vi "FPGA_BIDIR_Sensores_dobles.vi"() -> ()   [LabVIEW 2015]
uses:
  <vilib>/LabVIEW Targets/FPGA/cRIO/shared/nicrio_ModuleControls/nicrio_cRIO-9234_DataRatesRing2.ctl
  <vilib>/LabVIEW Targets/FPGA/cRIO/shared/nicrio_ModuleControls/nicrio_BasicConversionTime.ctl
  <vilib>/rvi/Emulation/niFpgaGetClockAttributes.vi
  <vilib>/rvi/Emulation/niFpgaSctlEmulationGetInTimedLoop.vi
  <vilib>/rvi/Emulation/niFpgaEmulationReportErrorSimple.vi
  <vilib>/rvi/Emulation/niFpgaProcessEmulError.vi
  <vilib>/rvi/eio/common/nirviEmuTemplateMethod_errors.vi
  <vilib>/rvi/Emulation/niFpgaCriticalErrorInLSC.vi
  <vilib>/rvi/eio/common/nirviEmuTemplatePropertySet_errors.vi
  <vilib>/rvi/interface/RandomDataEmulation/niFpgaRandomDataHandleErrors.vi
  <vilib>/eio/EIONode/EIONode.xnode
  <vilib>/eio/EIOPropertyNode/EIOPropertyNode.xnode
  <vilib>/rvi/DataTransferAndStorage/Container/XNode/niFpgaContainer.xnode
  <vilib>/rvi/interface/RandomDataEmulation/nirviRandomDataFpgaReadWriteTemplate.vi
  <vilib>/rvi/eio/common/nirviEmuTemplatePropertyGet_errors.vi
  <vilib>/rvi/eio/common/nirviEmuTemplatePropertyGet_noerrors.vi
  <vilib>/rvi/eio/common/nirviEmuTemplatePropertySet_noerrors.vi
panel:
  out "Numeric 2":i32
  out "WhlCnt1":fxp<+/-,24,-4> format="%.27g"
  in  "Offset_WS1":fxp<+/-,24,-4>=0.000999998301267624 format="%.27g"
  out "Rueda1?":i16
  out "WhlCnt2":fxp<+/-,24,-4> format="%.27g"
  out "Rueda2?":i16
  out "RuedaDetectada1?":bool
  out "RuedaDetectada2?":bool
  out "Parar":bool
  out "Nº Ruedas 1":i32
  out "NºRuedas 2":i32
  in  "Offset_WS2":fxp<+/-,24,-4>=0.000999998301267624 format="%.27g"
  in  "Cycles to Filter":u16=5
  in  "Canal cero WS1?":bool=TRUE
  in  "Canal cero WS2?":bool=TRUE
  in  "Conversion Time":T1
  in  "Count(mSec)":u32=2
  in  "Stop":bool
  out "Buffer Underflow":bool
  in  "Digital?":bool=TRUE
  out "medidas":fxp<+/-,24,4>[](array[numeric])
  out "Buffer Overflow":bool
  out "Error Out":errorcluster
  in  "Data Rate":T2=2 items=["51.200 kS/s (NI 9234)"=1, "25.600 kS/s (NI 9234)"=2, "17.067 kS/s (NI 9234)"=3, "12.800 kS/s (NI 9234)"=4, "10.240 kS/s (NI 9234)"=5, "8.533 kS/s (NI 9234)"=6, "7.314 kS/s (NI 9234)"=7, "6.400 kS/s (NI 9234)"=8, "5.689 kS/s (NI 9234)"=9, "5.120 kS/s (NI 9234)"=10, "4.654 kS/s (NI 9234)"=11, "4.267 kS/s (NI 9234)"=12, "3.938 kS/s (NI 9234)"=13, "3.657 kS/s (NI 9234)"=14, "3.413 kS/s (NI 9234)"=15, "3.200 kS/s (NI 9234)"=16, "3.012 kS/s (NI 9234)"=17, "2.845 kS/s (NI 9234)"=18, "2.695 kS/s (NI 9234)"=19, "2.560 kS/s (NI 9234)"=20, "2.438 kS/s (NI 9234)"=21, "2.328 kS/s (NI 9234)"=22, "2.226 kS/s (NI 9234)"=23, "2.133 kS/s (NI 9234)"=24, "2.048 kS/s (NI 9234)"=25, "1.969 kS/s (NI 9234)"=26, "1.896 kS/s (NI 9234)"=27, "1.829 kS/s (NI 9234)"=28, "1.765 kS/s (NI 9234)"=29, "1.707 kS/s (NI 9234)"=30, "1.652 kS/s (NI 9234)"=31]
  out "DC OK":bool
  in  "Fotocélula":bool
  out "Detector de\npresencia":bool
  out "Chassis Temperature":i16
  out "Direccion 0?":bool
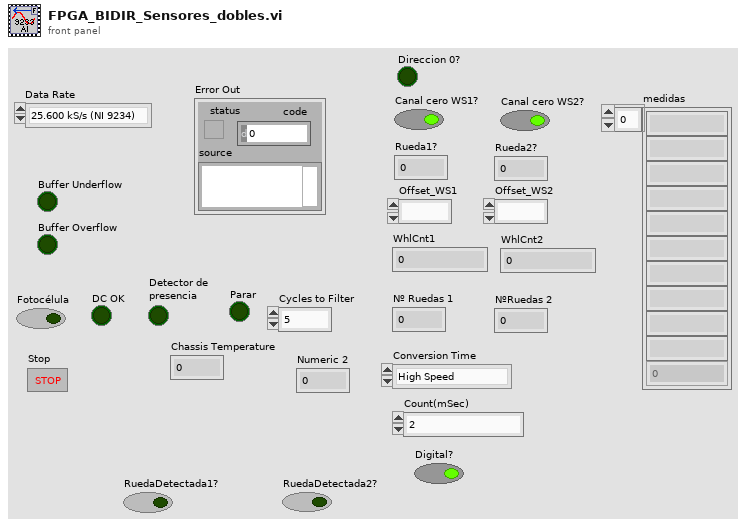
[diagram p1: front panel]
types:
  T1 = typedef "nicrio_BasicConversionTime.ctl" = enum8{"High Speed", "High Resolution"}
  T2 = typedef "nicrio_cRIO-9234_DataRatesRing2.ctl" = u8
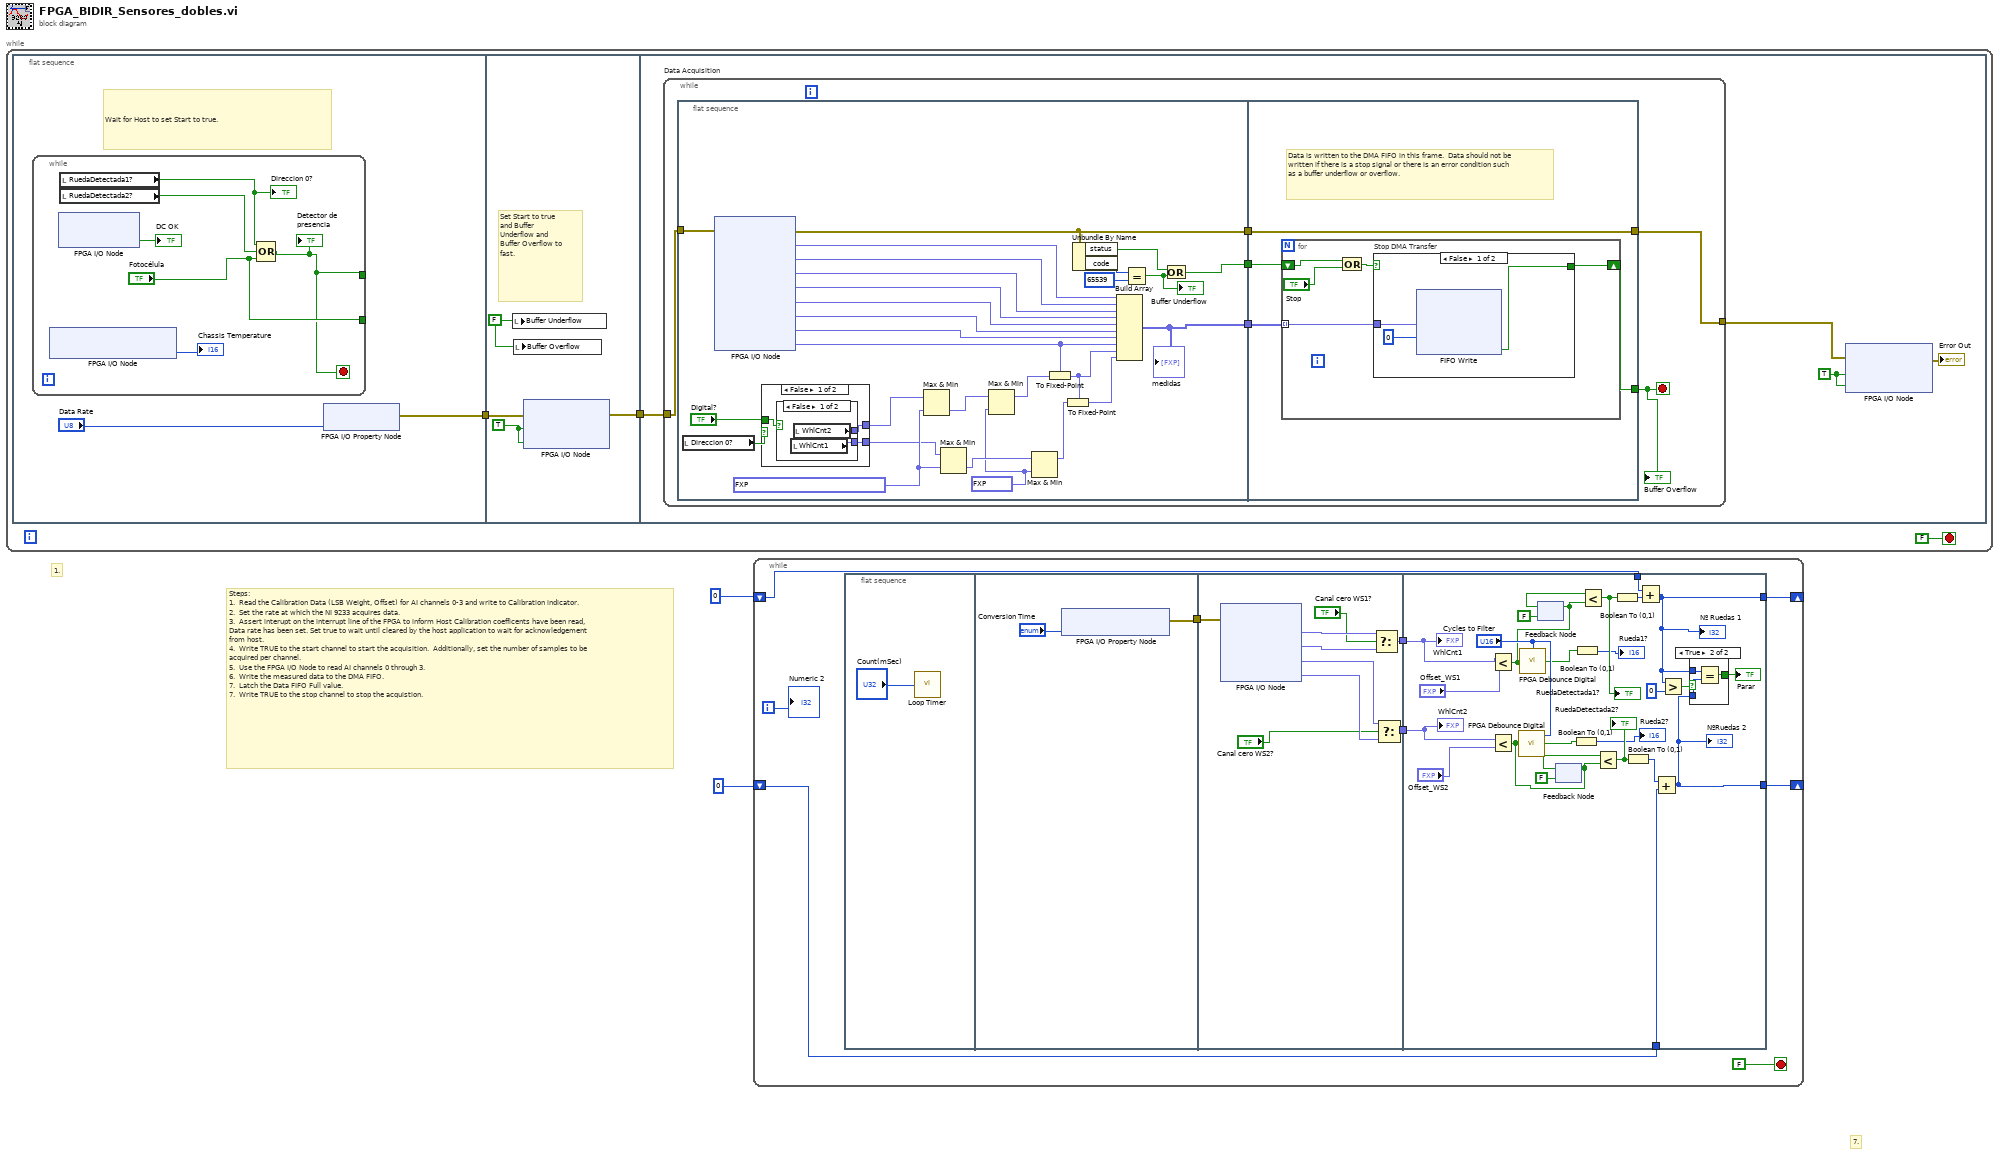
[diagram p0: block diagram]
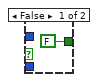
[diagram p2: hidden frame]
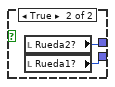
[diagram p3: hidden frame]
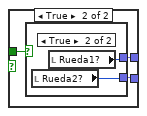
[diagram p4: hidden frame]
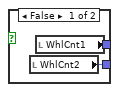
[diagram p5: hidden frame]
diagram:
  # "Steps: \n1.  Read the Calibration Data (LSB Weight, Offset) for AI channels 0-3 and write to Calibration indicator.\n2.  Set the rate at which the NI 9233 acquires data. \n3.  Assert interupt on the interrupt line of the FPGA to inform Host Calibration coefficents have been read, Data rate has been set. Set true to wait until cleared by the host application to wait for acknowledgement from host.\n4.  Write TRUE to the start channel to start the acquisition.  Additionally, set the number of samples to be acquired per channel.\n5.  Use the FPGA I/O Node to read AI channels 0 through 3. \n6.  Write the measured data to the DMA FIFO.\n7.  Latch the Data FIFO Full value.\n7.  Write TRUE to the stop channel to stop the acquistion."
  # "1."
  # "7."
  n1 = while {
    stop <- FALSE stop-if-true
    n2 = flat-sequence "MainSeq" {
      tunnel: [w7] -> w4
      tunnel: w4 -> [w16]
      tunnel: [w15] -> w3
      tunnel: w3 -> [w21]
      frame #0 {
        # "Wait for Host to set Start to true."
        n3 = while "initWait" {
          tunnel: ["Fotocélula"] -> _
          tunnel: [w9] -> _
          stop <- w9 stop-if-true
          n4 = xnode "FPGA I/O Node"() -> ("Chassis Temperature"=→"Chassis Temperature":i16)  [unwired: 1 in, 1 out]
          n5 = xnode "FPGA I/O Node"() -> ("Mod3/DI2"=→"DC OK":bool)  [unwired: 2 in, 2 out]
          n6 = local read "RuedaDetectada1?"() -> (w8:bool)
          "Direccion 0?" <- w8
          n7 = local read "RuedaDetectada2?"() -> (w10:bool)
          n8 = Compound Arithmetic op=OR(w8, w10, "Fotocélula") -> (w9:bool)
          "Detector de\npresencia" <- w9
        }
        n9 = xnode "FPGA I/O Property Node"("Data Rate"="Data Rate") -> ("error out"=w7:errorcluster)  [unwired: 2 in, 1 out]
      }
      frame #1 {
        w14 = TRUE
        w17 = FALSE ("Late? (Latched)")
        # "Set Start to true and Buffer Underflow and Buffer Overflow to fast."
        n10 = local write "Buffer Underflow"(w17) -> ()
        n11 = local write "Buffer Overflow"(w17) -> ()
        n12 = xnode "FPGA I/O Node"("error in"=w16, "Mod1/Start"=w14, "Mod2/Start"=w14) -> ("error out"=w15:errorcluster)  [unwired: 2 in, 2 out]
      }
      frame #2 {
        w18 = TRUE
        n13 = while "Data Acquisition" {
          tunnel: w21 -> [w25]
          tunnel: [w24] -> w19
          stop <- w22 stop-if-true
          n14 = flat-sequence "Data Acquisition Sequence" {
            tunnel: [w55] -> w27
            tunnel: [w49] -> w26
            tunnel: w25 -> [w54]
            tunnel: [w53] -> w23
            tunnel: w27 -> [w73]
            tunnel: w26 -> [w72]
            tunnel: [w71] -> w22
            tunnel: [w70] -> w24
            tunnel: w23 -> [w70]
            frame #0 {
              w32 = fxp<+/-,44,16> -0.03125 ("y")
              w34 = fxp<+/-,44,16> 0.0312499962747097 ("y")
              n15 = local read "Direccion 0?"() -> (w46:bool)
              n16 = xnode "FPGA I/O Node"("error in"=w54) -> ("error out"=w53:errorcluster, "Mod1/AI0"=w43:fxp<+/-,24,4>, "Mod1/AI1"=w42:fxp<+/-,24,4>, "Mod1/AI2"=w41:fxp<+/-,24,4>, "Mod1/AI3"=w40:fxp<+/-,24,4>, "Mod2/AI0"=w39:fxp<+/-,24,4>, "Mod2/AI1"=w38:fxp<+/-,24,4>, "Mod2/AI2"=w37:fxp<+/-,24,4>, "Mod2/AI3"=w36:fxp<+/-,24,4>)  [unwired: 8 in, 8 out]
              n17 = case shown="False" w46 {
                tunnel: "Digital?" -> [w58 w65]
                tunnel: [w57 w64] -> w30
                tunnel: [w56 w63] -> w29
                frame False {
                  n18 = case shown="False" w58 {
                    tunnel: [w60 w62] -> w57
                    tunnel: [w59 w61] -> w56
                    frame False {
                      n19 = local read "WhlCnt1"() -> (w59:fxp<+/-,24,-4>)
                      n20 = local read "WhlCnt2"() -> (w60:fxp<+/-,24,-4>)
                    }
                    frame True {
                      n21 = local read "Rueda2?"() -> (w62:i16)
                      n22 = local read "Rueda1?"() -> (w61:i16)
                    }
                  }
                }
                frame True {
                  n23 = case shown="True" w65 {
                    tunnel: [w67 w69] -> w64
                    tunnel: [w66 w68] -> w63
                    frame False {
                      n24 = local read "WhlCnt2"() -> (w66:fxp<+/-,24,-4>)
                      n25 = local read "WhlCnt1"() -> (w67:fxp<+/-,24,-4>)
                    }
                    frame True {
                      n26 = local read "Rueda2?"() -> (w68:i16)
                      n27 = local read "Rueda1?"() -> (w69:i16)
                    }
                  }
                }
              }
              n28 = Max & Min(x=w30, y=w34) -> (min(x,y)=w33:fxp<+/-,44,16>)  [unwired: 1 out]
              n29 = Max & Min(x=w29, y=w34) -> (min(x,y)=w35:fxp<+/-,44,16>)  [unwired: 1 out]
              n30 = Max & Min(x=w33, y=w32) -> (max(x,y)=w31:fxp<+/-,44,16>)  [unwired: 1 out]
              n31 = Max & Min(x=w35, y=w32) -> (max(x,y)=w28:fxp<+/-,44,16>)  [unwired: 1 out]
              n32 = To Fixed-Point(fixed-point type=w36, number=w31) -> (fixed-point=w45:fxp<+/-,24,4>)
              n33 = To Fixed-Point(fixed-point type=w45, number=w28) -> (fixed-point=w44:fxp<+/-,24,4>)
              n34 = Unbundle By Name(w53) -> ("status"=w48:bool, "code"=w52:i32)
              n35 = Build Array(w43, w42, w41, w40, w39, w38, w37, w36, w45, w44) -> (w55:fxp<+/-,24,4>[])
              "medidas" <- w55
              n36 = Equal?(x=w52, y=65539) -> (x = y?=w50:bool)
              "Buffer Underflow" <- w50
              n37 = Or(x=w48, y=w50) -> (x .or. y?=w49:bool)
            }
            frame #1 {
              # "Data is written to the DMA FIFO in this frame.  Data should not be written if there is a stop signal or there is an error condition such as a buffer underflow or overflow."
              n38 = for "DMAWriteLoop" {
                tunnel: w73 -> [w78] mode=indexing
                shift-right: [w77] -> w71
                shift-left: w72 -> [w76]
                n39 = Compound Arithmetic op=OR(w76, "Stop") -> (w75:bool)
                n40 = case "Stop DMA Transfer" shown="False" w75 {
                  selector: w75 -> [_ w82]
                  tunnel: w78 -> [w79 _]
                  tunnel: [w81 w82] -> w77
                  frame False {
                    n41 = xnode ("FIFO Write")("Element"=w79, "Timeout"=0) -> ("Timed Out?"=w81:bool)  [unwired: 1 in, 1 out]
                  }
                  frame True {
                  }
                }
              }
            }
          }
          "Buffer Overflow" <- w22
        }
        n42 = xnode "FPGA I/O Node"("error in"=w19, "Mod1/Stop"=w18, "Mod2/Stop"=w18) -> ("error out"=→"Error Out":errorcluster)  [unwired: 2 in, 2 out]
      }
    }
  }
  n43 = while {
    shift-right: [w88] -> _
    shift-left: 0 -> [w87]
    shift-right: [w85] -> _
    shift-left: 0 -> [w86]
    i -> [w84]
    stop <- FALSE stop-if-true
    n44 = flat-sequence {
      tunnel: [w93] -> w90
      tunnel: [w103] -> w91
      tunnel: w90 -> [w97]
      tunnel: [w100] -> w89
      tunnel: w91 -> [w129]
      tunnel: w89 -> [w127]
      tunnel: [w117] -> w88
      tunnel: w87 -> [w124]
      tunnel: w86 -> [w122]
      tunnel: [w116] -> w85
      frame #0 {
        n45 = call "Loop Timer"("Count(mSec)"="Count(mSec)") -> ()  [unwired: 1 out]
      }
      frame #1 {
        n46 = xnode "FPGA I/O Property Node"("Conversion Time"="Conversion Time") -> ("error out"=w93:errorcluster)  [unwired: 2 in, 1 out]
      }
      frame #2 {
        n47 = xnode "FPGA I/O Node"("error in"=w97) -> ("Mod4/AI0"=w102:fxp<+/-,24,-4>, "Mod4/AI1"=w101:fxp<+/-,24,-4>, "Mod4/AI2"=w99:fxp<+/-,24,-4>, "Mod4/AI3"=w98:fxp<+/-,24,-4>)  [unwired: 4 in, 5 out]
        n48 = Select(t=w102, s="Canal cero WS1?", f=w101) -> (s? t:f=w103:fxp<+/-,24,-4>)
        n49 = Select(t=w99, s="Canal cero WS2?", f=w98) -> (s? t:f=w100:fxp<+/-,24,-4>)
      }
      frame #3 {
        n50 = Less?(x=w129, y="Offset_WS1") -> (x < y?=w107:bool)
        n51 = Less?(x=w127, y="Offset_WS2") -> (x < y?=w105:bool)
        n52 = call "FPGA Debounce Digital.vi"("Input Signal"=w105, "Cycles to Filter"="Cycles to Filter") -> ("Output Filtered Signal"=w104:bool)
        n53 = call "FPGA Debounce Digital.vi"("Input Signal"=w107, "Cycles to Filter"="Cycles to Filter") -> ("Output Filtered Signal"=w106:bool)
        n54 = feedback-in #1(w107) -> ()
        n55 = feedback #1(FALSE) -> (w125:bool)
        n56 = feedback #2(FALSE) -> (w118:bool)
        n57 = feedback-in #2(w105) -> ()
        n58 = Boolean To (0,1)(Boolean=w104) -> (0, 1=→"Rueda2?":i16)
        n59 = Boolean To (0,1)(Boolean=w106) -> (0, 1=→"Rueda1?":i16)
        n60 = Less?(x=w125, y=w107) -> (x < y?=w113:bool)
        "RuedaDetectada1?" <- w113
        n61 = Less?(x=w118, y=w105) -> (x < y?=w112:bool)
        "RuedaDetectada2?" <- w112
        n62 = Boolean To (0,1)(Boolean=w113) -> (0, 1=w109:i16)
        n63 = Boolean To (0,1)(Boolean=w112) -> (0, 1=w114:i16)
        n64 = Add(x=w124, y=w109) -> (x+y=w117:i32)
        "Nº Ruedas 1" <- w117
        n65 = Add(x=w114, y=w122) -> (x+y=w116:i32)
        "NºRuedas 2" <- w116
        n66 = Greater?(x=w117, y=i64 0) -> (0:w119:bool)
        n67 = case shown="True" w119 {
          tunnel: w116 -> [_ w133]
          tunnel: w117 -> [_ w132]
          tunnel: [FALSE w131] -> w121
          frame False {
          }
          frame True {
            n68 = Equal?(x=w132, y=w133) -> (x = y?=w131:bool)
          }
        }
        "Parar" <- w121
        "WhlCnt1" <- w129
        "WhlCnt2" <- w127
      }
    }
    "Numeric 2" <- w84
  }
